vi "Get Table Configuration.vi"(8 "error in (no error)":errorcluster, 11 "Panel Form Controller Configuration in":refnum<class "Panel Form Controller Configuration.lvclass">) -> (0 "error out":errorcluster, 2 "Table Configuration":refnum<class "Table Configuration Interface.lvclass">, 3 "Panel Form Controller Configuration out":refnum<class "Panel Form Controller Configuration.lvclass">)   [LabVIEW 2020]
uses:
  Panel Form Controller Configuration.lvclass
  Database OOP/Table Libraries/Table Configuration Interface/Table Configuration Interface.lvclass
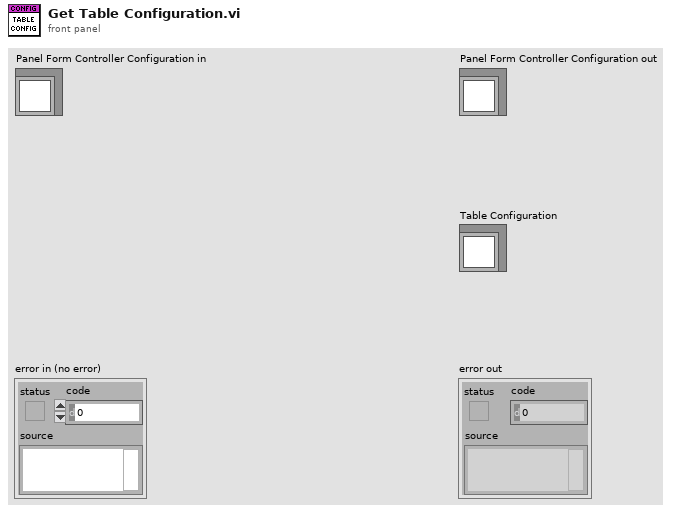
[diagram p1: front panel]
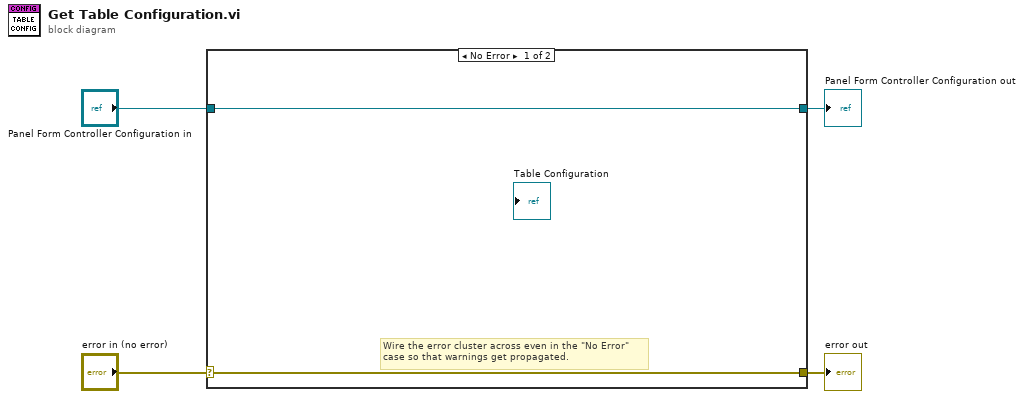
[diagram p0: block diagram]
diagram:
  n1 = case shown="No Error" "error in (no error)" {
    selector: "error in (no error)" -> [w5 w8]
    tunnel: [w5 w8] -> w3
    tunnel: [w6 w7] -> w1
    tunnel: "Panel Form Controller Configuration in" -> [w6 w7]
    frame No Error {
      # "Wire the error cluster across even in the \"No Error\"\ncase so that warnings get propagated."
    }
    frame Error {
    }
  }
  "error out" <- w3
  "Panel Form Controller Configuration out" <- w1
